vi "updatedAt.get.vi"(8 "error in (no error)":errorcluster, 11 "Run in":refnum<class "Run.lvclass">) -> (0 "error out":errorcluster, 2 "updatedAt":timestamp format="%<%x %.3X>T", 3 "Run out":refnum<class "Run.lvclass">)   [LabVIEW 2020, in "Run.lvclass"]
uses:
  Run.lvclass
  Run.lvclass/Run.ctl
  Nominal Client/Nominal Client.lvclass
  3fa23586-c96c-44de-800b-8ec637a95f2c.vi
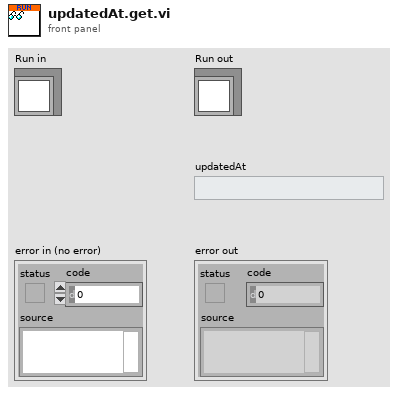
[diagram p1: front panel]
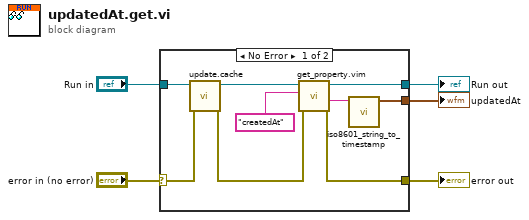
[diagram p0: block diagram]
diagram:
  n1 = case shown="No Error" "error in (no error)" {
    selector: "error in (no error)" -> [w14 w16]
    tunnel: "Run in" -> [w13 w15]
    tunnel: [w8 w16] -> w3
    tunnel: [w7 _] -> w2
    tunnel: [w6 w15] -> w1
    frame No Error {
      n2 = call "update.cache.vi"("error in"=w14, "Run in"=w13) -> ("error out"=w9:errorcluster, "Run out"=w10:refnum<class "Run.lvclass">)  [unwired: 8 in]
      n3 = call "get_property.vim"("error in"=w9, "Property Name"="createdAt", "Run in"=w10) -> ("error out"=w8:errorcluster, "Value"=w11:string, "Run out"=w6:refnum<class "Run.lvclass">)  [unwired: 6 in]
      n4 = call "iso8601_string_to_timestamp.vi"("ISO8601 Timestamp String"=w11) -> ("Time Stamp"=w7:timestamp)  [unwired: 9 in, 1 out]
    }
    frame Error {
    }
  }
  "error out" <- w3
  "Run out" <- w1
  "updatedAt" <- w2
